vi "acquire and process data.vi"(0 "connection ID":refnum<k5>, 7 "Reset":bool, 9 "Log Data":bool, 11 "error in":errorcluster, 12 "method":T1={"sampling interval"=0.1, "samples to average"=1, "data interval"=0.0, "stream data"=FALSE, "file path"=refnum, "command"={"command"=enum."Idle", "start time (ms)"=0, "Channel Indices"=[], "Scans per Sample"=1}} {"command"."Scans per Sample" min=1; "data interval" format="%.2f"; "samples to average" min=1 step=1; "sampling interval" format="%.2f"}) -> (2 "samples":u32, 4 "data out":sgl[][](array[numeric]) format="%.5f", 6 "last reading":sgl[](array[numeric]) format="%.2f", 8 "first derivative":sgl[](array[numeric]) format="%.2f", 10 "backlog":u32, 13 "Time":dbl[](array[numeric]) format="%.2f", 14 "Status":bool, 15 "error out":errorcluster)   [LabVIEW 2019]
uses:
  DAC apps/support/method.ctl
  DataServer/command.ctl
  DataServer/command cluster.ctl
panel:
  # "s"
  # "s"
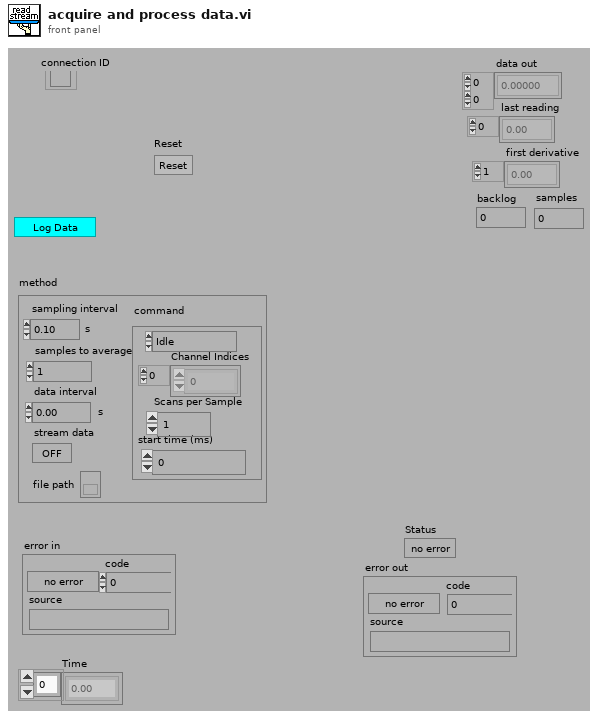
[diagram p1: front panel]
types:
  T1 = typedef "method.ctl" = cluster{"sampling interval":sgl, "samples to average":u32, "data interval":sgl, "stream data":bool, "file path":refnum<file>, "command":T2}
  T2 = typedef "command cluster.ctl" = cluster{"command":T3, "start time (ms)":u32, "Channel Indices":i32[], "Scans per Sample":i32}
  T3 = typedef "command.ctl" = enum16{"Idle", "Send Data", "Send 1 Scan", "Logoff"}
  T4 = typedef "data send.ctl" = cluster{"voltage data":sgl[], "scan backlog":u32, "seconds since 1904":dbl, "arbitrary scans":i32}
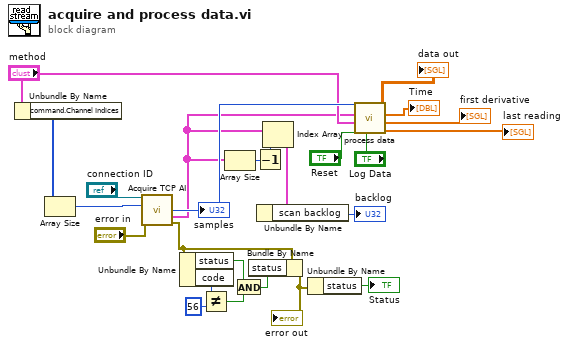
[diagram p0: block diagram]
diagram:
  n1 = Unbundle By Name("method") -> ("command.Channel Indices"=w9:i32[])
  n2 = Array Size(array=w9) -> (size(s)=w8:i32)
  n3 = call "Acquire TCP AI.vi"("connection ID"="connection ID", "channels"=w8, "error in"="error in") -> ("samples"=w11:u32, "data array"=w7:T4[], "error out"=w12:errorcluster)  [unwired: 8 in, 2 out]
  "samples" <- w11
  n4 = Unbundle By Name(w12) -> ("status"=w22:bool, "code"=w23:i32)
  n5 = Not Equal?(x=w23, y=56) -> (x != y?=w21:bool)
  n6 = Array Size(array=w7) -> (size(s)=w6:i32)
  n7 = And(x=w22, y=w21) -> (x .and. y?=w20:bool)
  n8 = Bundle By Name(cluster=w12, "status"=w20) -> (w13:errorcluster)
  "error out" <- w13
  n9 = Decrement(x=w6) -> (x-1=w5:i32)
  n10 = Index Array(array=w7, index=w5) -> (element=w15:T4)
  n11 = Unbundle By Name(w15) -> ("scan backlog"=→"backlog":u32)
  n12 = Unbundle By Name(w13) -> ("status"=→"Status":bool)
  n13 = call "process data.vi"("Log Data"="Log Data", "Reset"="Reset", "method"="method", "data array"=w7, "successes"=w11) -> ("last reading"=→"last reading":sgl[], "first derivative"=→"first derivative":sgl[], "Time"=→"Time":dbl[], "scaled data out"=→"data out":sgl[][])  [unwired: 3 in]
